vi "Thingworx_ParseJSON.vi"(11 "Comm":T2) -> (2 "Table Control":string[][](table)=[["test", "test", "STRING"]], 3 "Data":T1(array[cluster]))   [LabVIEW 2019]
panel:
  out "Thing":string
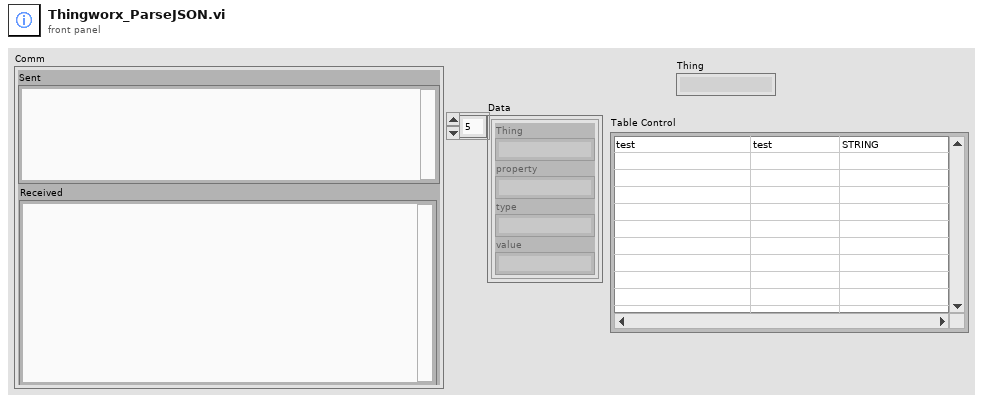
[diagram p1: front panel]
types:
  T1 = cluster{"Thing":string, "property":string, "type":string, "value":string}[]
  T2 = cluster{"url":string, "sent headers":string, "sent body":string, "headers":string, "body":string, "Sent":string, "Received":string}
  T3 = cluster{"Thing":string, "property":string, "type":string, "value":string}
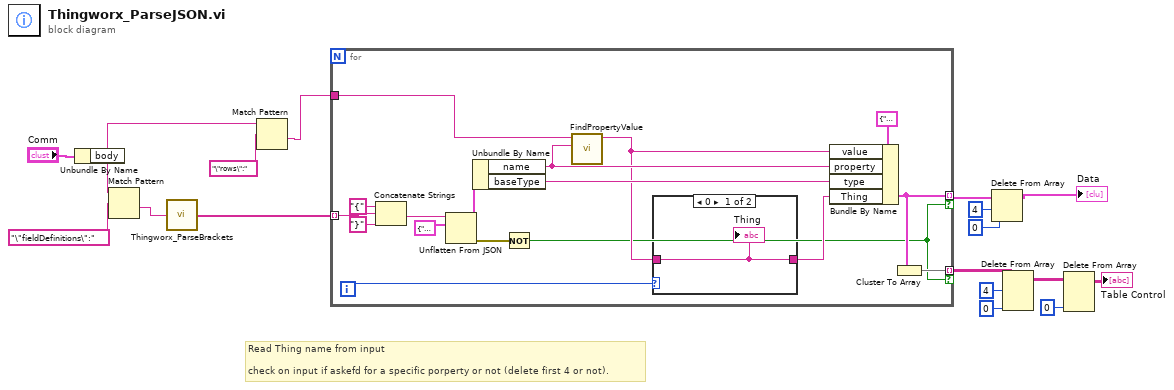
[diagram p0: block diagram]
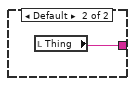
[diagram p2: hidden frame]
diagram:
  # "Read Thing name from input\n\ncheck on input if askefd for a specific porperty or not (delete first 4 or not)."
  n1 = Unbundle By Name("Comm") -> ("body"=w12:string)
  n2 = Match Pattern(string=w12, regular expression="\"fieldDefinitions\":") -> (after substring=w16:string)  [unwired: 1 in, 3 out]
  n3 = call "Thingworx_ParseBrackets.vi"("body"=w16) -> ("In Brackets"=w14:string[])
  n4 = Match Pattern(string=w12, regular expression="\"rows\":") -> (after substring=w11:string)  [unwired: 1 in, 3 out]
  n5 = for {
    tunnel: [w20] -> w10 mode=indexing if=w18
    tunnel: w14 -> [w30] mode=indexing
    tunnel: w11 -> [w25]
    tunnel: [w19] -> w4 mode=indexing if=w18
    i -> [w24]
    n6 = Concatenate Strings("{" ("string"), w30, "}" ("string")) -> (w34:string)
    n7 = Unflatten From JSON(JSON string=w34, type and defaults=cluster{"name":string, "baseType":string} {"name"="", "baseType"=""}) -> (value=w27:cluster{"name":string, "baseType":string}, error out=w28:errorcluster)  [unwired: 5 in]
    n8 = Unbundle By Name(w27) -> ("name"=w22:string, "baseType"=w26:string)
    n9 = Not(x=w28) -> (.not. x?=w18:bool)
    n10 = call "FindPropertyValue.vi"("property"=w22, "rows"=w25) -> ("value"=w21:string)  [unwired: 9 in]
    n11 = case shown="0" w24 {
      tunnel: [w35 w36] -> w23
      tunnel: w21 -> [w35 _]
      frame 0 {
        "Thing" <- w35
      }
      frame Default {
        n12 = local read "Thing"() -> (w36:string)
      }
    }
    n13 = Bundle By Name(cluster=T3 {"Thing"="", "property"="", "type"="LONG", "value"=""} ("Property In"), "value"=w21, "property"=w22, "type"=w26, "Thing"=w23) -> (w20:T3)
    n14 = Cluster To Array(cluster=w20) -> (array=w19:string[])
  }
  n15 = Delete From Array(array=w10, length=4, index=0) -> (array with subset deleted=→"Data":T1)  [unwired: 1 out]
  n16 = Delete From Array(array=w4, length=4, index (row)=0 ("index")) -> (array with subset deleted=w3:string[][])  [unwired: 1 in, 1 out]
  n17 = Delete From Array(array=w3, index (col)=0 ("disabled index (col)")) -> (array with subset deleted=→"Table Control":string[][])  [unwired: 2 in, 1 out]
